vi "Write Channel Info.vi"(6 "DataType":T1, 7 "Read or Write":string, 8 "error in (no error)":errorcluster, 9 "URL":string, 10 "Name":string, 11 "Channel in":refnum<class "Channel.lvclass">) -> (0 "error out":errorcluster, 3 "Channel out":refnum<class "Channel.lvclass">)   [LabVIEW 2017, in "Channel.lvlib" / "Channel.lvclass"]
uses:
  Channel.lvclass
  <vilib>/Utility/Data Type/Type Definitions/Data Type.ctl
  Channel.lvclass/Channel.ctl
  <vilib>/Utility/Data Type/NI_Data Type.lvlib
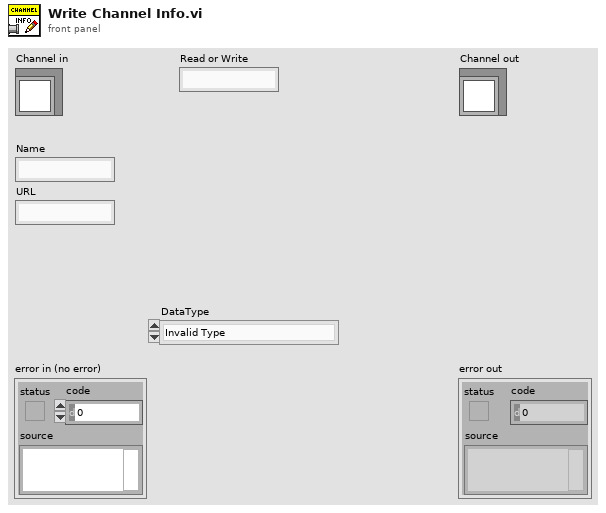
[diagram p1: front panel]
types:
  T1 = typedef "NI_Data Type.lvlib/Data Type.ctl" = enum8{"Invalid Type", "Void", "I8", "I16", "I32", "I64", "U8", "U16", "U32", "U64", "Single Float", "Double Float", "Extended Float", "Single Complex", "Double Complex", "Extended Complex", "Enum U8", "Enum U16", "Enum U32", "Enum U64", "Single Float With Unit", "Double Float With Unit", "Extended Float With Unit", "Single Complex with Unit", "Double Complex with Unit", "Extended Complex with Unit", "Boolean", "String", "Path", "Picture", "Tag", "Array", "Cluster", "Variant", "LV Variant", "Waveform", "Timestamp", "Digital Waveform", "Digital Data", "ExpressData", "Refnum", "External Data", "VI", "Poly VI", "LabVIEW Class Instance", "Fixed Point"}
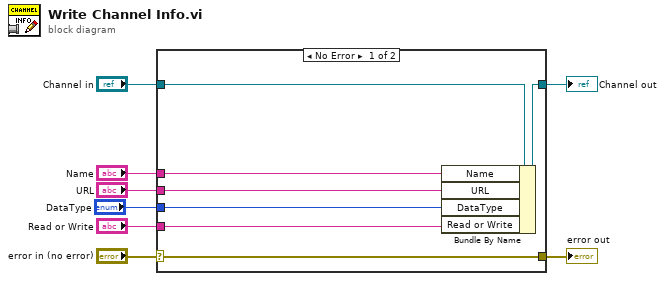
[diagram p0: block diagram]
diagram:
  n1 = case shown="No Error" "error in (no error)" {
    selector: "error in (no error)" -> [w15 w16]
    tunnel: [w15 w16] -> w7
    tunnel: [w13 w17] -> w5
    tunnel: "Channel in" -> [w14 w17]
    tunnel: "Name" -> [w12 _]
    tunnel: "URL" -> [w11 _]
    tunnel: "Read or Write" -> [w10 _]
    tunnel: "DataType" -> [w9 _]
    frame No Error {
      n2 = Bundle By Name(cluster=w14, "Name"=w12, "URL"=w11, "DataType"=w9, "Read or Write"=w10) -> (w13:refnum<class "Channel.lvclass">)
    }
    frame Error {
    }
  }
  "error out" <- w7
  "Channel out" <- w5
